vi "Cannon Modifications.vi"(1 "Cannon Info":T1, 2 "InTake Max":bool) -> (0 "Cannon Info":T1)   [LabVIEW 2013]
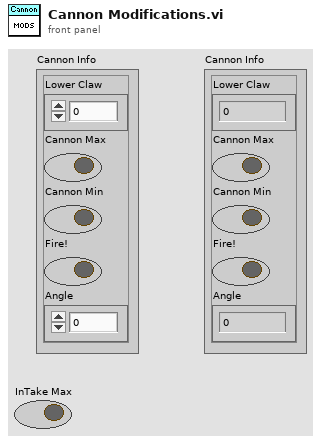
[diagram p1: front panel]
types:
  T1 = cluster{"Lower Claw":dbl, "Cannon Max":bool, "Cannon Min":bool, "Fire!":bool, "Angle":dbl}
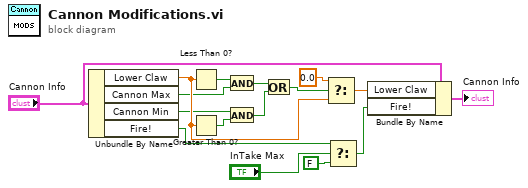
[diagram p0: block diagram]
diagram:
  n1 = Unbundle By Name("Cannon Info") -> ("Lower Claw"=w10:dbl, "Cannon Max"=w3:bool, "Cannon Min"=w4:bool, "Fire!"=w9:bool)
  n2 = Less Than 0?(x=w10) -> (x < 0?=w12:bool)
  n3 = Greater Than 0?(x=w10) -> (x > 0?=w14:bool)
  n4 = And(x=w12, y=w3) -> (x .and. y?=w13:bool)
  n5 = And(x=w4, y=w14) -> (x .and. y?=w1:bool)
  n6 = Or(x=w13, y=w1) -> (x .or. y?=w11:bool)
  n7 = Select(t=0.0, s=w11, f=w10) -> (s? t:f=w8:dbl)
  n8 = Select(t=w9, s="InTake Max", f=FALSE) -> (s? t:f=w7:bool)
  n9 = Bundle By Name(cluster="Cannon Info", "Lower Claw"=w8, "Fire!"=w7) -> (→"Cannon Info":T1)
